vi "DSF.Shared.Timing.Is Active Cycle.vi"(10 "iteration":u64=1, 11 "Timing in":refnum<class "DSF.Shared.Timing.lvclass">) -> (2 "active?":bool, 3 "Timing out":refnum<class "DSF.Shared.Timing.lvclass">)   [LabVIEW 2017, in "DSF.Shared.lvlib" / "DSF.Shared.Timing.lvclass"]
uses:
  DSF.Shared.Timing.lvclass
  DSF.Shared.Timing.lvclass/DSF.Shared.Timing.ctl
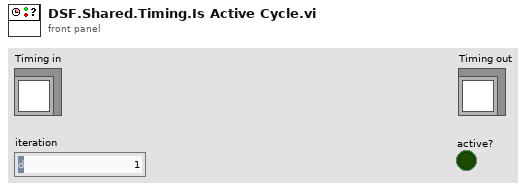
[diagram p1: front panel]
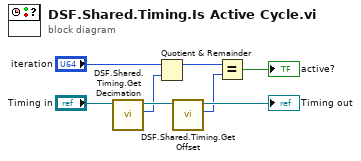
[diagram p0: block diagram]
diagram:
  n1 = call "DSF.Shared.Timing.Get Decimation.vi"("Timing in"="Timing in") -> ("Decimation"=w3:u64, "Timing out"=w7:refnum<class "DSF.Shared.Timing.lvclass">)  [unwired: 9 in]
  n2 = Quotient & Remainder(x="iteration", y=w3) -> (x-y*floor(x/y)=w6:u64)  [unwired: 1 out]
  n3 = call "DSF.Shared.Timing.Get Offset.vi"("Timing in"=w7) -> ("Offset"=w4:u64, "Timing out"=→"Timing out":refnum<class "DSF.Shared.Timing.lvclass">)  [unwired: 9 in]
  n4 = Equal?(x=w6, y=w4) -> (x = y?=→"active?":bool)
